vi "Mixer.Read Level.vi"(0 "baseURL":string="http://169.254.128.32/datastore/", 11 "error in (no error)":errorcluster) -> (4 "baseURL out":string="http://169.254.128.32/datastore/", 8 "value":dbl, 15 "error out":errorcluster)   [LabVIEW 2020]
uses:
  <vilib>/httpClient/LabVIEWHTTPClient.lvlib
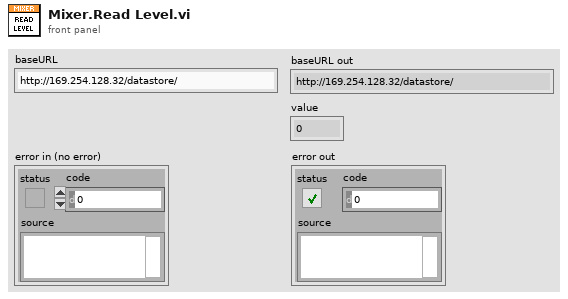
[diagram p1: front panel]
types:
  T1 = typedef "LabVIEWHTTPClient.lvlib/ClientHandle.ctl" = refnum<k1>
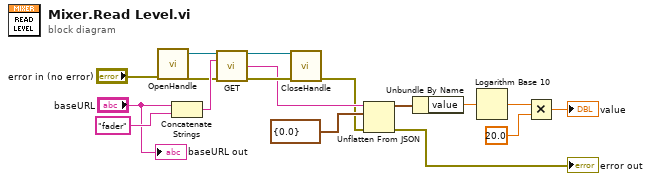
[diagram p0: block diagram]
diagram:
  n1 = call <vilib>:"OpenHandle.vi"("error in (no error)"="error in (no error)") -> ("client handle out"=w13:T1, "error out"=w12:errorcluster)  [unwired: 13 in]
  n2 = Concatenate Strings("baseURL", "fader") -> (w14:string)
  n3 = call <vilib>:"GET.vi"("client handle"=w13, "url"=w14, "error in (no error)"=w12) -> ("client handle out"=w11:T1, "body"=w9:string, "error out"=w10:errorcluster)  [unwired: 9 in, 1 out]
  n4 = call <vilib>:"CloseHandle.vi"("client handle"=w11, "error in (no error)"=w10) -> ("error out"=w6:errorcluster)  [unwired: 13 in]
  n5 = Unflatten From JSON(JSON string=w9, type and defaults=cluster{"value":dbl} {"value"=0.0}, error in (no error)=w6) -> (value=w7:cluster{"value":dbl}, error out=→"error out":errorcluster)  [unwired: 4 in]
  n6 = Unbundle By Name(w7) -> ("value"=w4:dbl)
  n7 = Logarithm Base 10(1:w4) -> (0:w3:dbl)
  n8 = Multiply(x=w3, y=20.0) -> (x*y=→"value":dbl)
  "baseURL out" <- "baseURL"
